vi "Write Attributes.vi"(4 "Actor Ref":refnum<vi>, 5 "Alias":string, 6 "Creator Attributes":refnum<class "Attributes.lvclass">, 7 "Unified Msg Set":T1, 9 "Queue of Self Attributes":refnum<queue>, 10 "Queue of Error":refnum<queue>, 11 "TEMPLATE Actor in":refnum<class "TEMPLATE Actor.lvclass">) -> (0 "Error out":errorcluster, 3 "TEMPLATE Actor out":refnum<class "TEMPLATE Actor.lvclass">)   [LabVIEW 2020, in "_Template.lvlib" / "Templates.lvlib" / "TEMPLATE Actor.lvlib" / "TEMPLATE Actor.lvclass"]
uses:
  TEMPLATE Actor.lvclass
  C:/git/jettl/src/jettl/jettl/Actor/Actor/Actor.lvclass
  jettl/jettl/Attributes/Attributes/Attributes.lvclass
  jettl/jettl/Actor/Msg Set.ctl
  jettl/jettl/Msg/Msg.lvclass
  TEMPLATE Actor.lvclass/TEMPLATE Actor.ctl
  jettl/jettl/Actor/Actor/Actor.lvclass
  jettl/jettl/Actor/Actor.lvlib
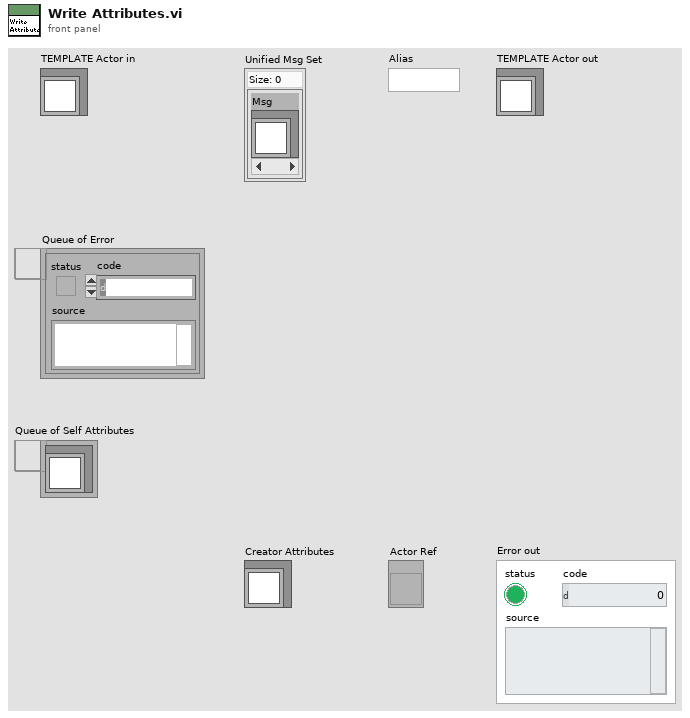
[diagram p1: front panel]
types:
  T1 = typedef "jettl.lvlib/Actor.lvlib/Msg Set.ctl" = set{refnum<class "Msg.lvclass">}
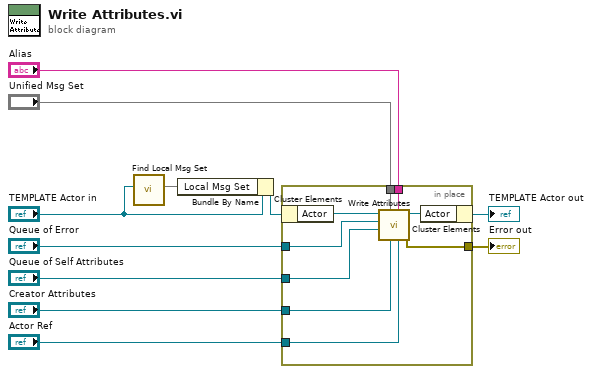
[diagram p0: block diagram]
diagram:
  n1 = call "Find Local Msg Set.vi"("Appliction Ref"="TEMPLATE Actor in") -> ("Local Msg Set"=w1:T1)  [unwired: 10 in]
  n2 = Bundle By Name(cluster="TEMPLATE Actor in", "Local Msg Set"=w1) -> (w2:refnum<class "TEMPLATE Actor.lvclass">)
  n3 = in-place {
    in-place-border: "Queue of Error" -> [w18]
    in-place-border: "Queue of Self Attributes" -> [w17]
    in-place-border: "Unified Msg Set" -> [w16]
    in-place-border: "Alias" -> [w15]
    in-place-border: "Creator Attributes" -> [w14]
    in-place-border: "Actor Ref" -> [w13]
    in-place-border: [w12] -> w4
    n4 = in-place-cluster #1(w2) -> ("Actor"=w20:refnum<class "Actor.lvclass">)
    n5 = call-dynamic "Write Attributes.vi"("Actor Ref"=w13, "Alias"=w15, "Creator Attributes"=w14, "Unified Msg Set"=w16, "Queue of Self Attributes"=w17, "Queue of Error"=w18, "Actor in"=w20) -> ("Error out"=w12:errorcluster, "Actor out"=w19:refnum<class "Actor.lvclass">)  [unwired: 3 in]
    n6 = in-place-cluster #1("Actor"=w19) -> (→"TEMPLATE Actor out":refnum<class "TEMPLATE Actor.lvclass">)
  }
  "Error out" <- w4
